vi "test-CoordinateSystem-checkTransform3dConvert.vi"(8 "COORDINATE_SYSTEM_TO":T1={"Rotation"={"Q_quaternion"={"R"=1.0, "V"=[0.0, 0.0, 0.0]}}}, 9 "COORDINATE_SYSTEM_FROM":T1={"Rotation"={"Q_quaternion"={"R"=1.0, "V"=[0.0, 0.0, 0.0]}}}, 10 "Transform3D_TO":T4={"TRANSLATION3D"={"X"=0.0, "Y"=0.0, "Z"=0.0}, "ROTATION3D"={"Q_quaternion"={"R"=1.0, "V"=[0.0, 0.0, 0.0]}}, "XF"=FALSE} {"TRANSLATION3D"."Z" format="%14.3f"; "TRANSLATION3D"."Y" format="%14.3f"; "TRANSLATION3D"."X" format="%14.3f"}, 11 "Transform3D_FROM":T4={"TRANSLATION3D"={"X"=0.0, "Y"=0.0, "Z"=0.0}, "ROTATION3D"={"Q_quaternion"={"R"=1.0, "V"=[0.0, 0.0, 0.0]}}, "XF"=FALSE} {"TRANSLATION3D"."Z" format="%14.3f"; "TRANSLATION3D"."Y" format="%14.3f"; "TRANSLATION3D"."X" format="%14.3f"}) -> (3 "All tests passed":bool)   [LabVIEW 2019]
uses:
  <vilib>/Rock Robotics/WPI/ThirdParty/JAS_Junk/TrajLib/TypeDef/TRANSFORM3D.ctl
  <vilib>/Rock Robotics/WPI/ThirdParty/JAS_Junk/TrajLib/TypeDef/TRANSLATION3D.ctl
  <vilib>/Rock Robotics/WPI/ThirdParty/JAS_Junk/TrajLib/TypeDef/ROTATION3D.ctl
  <vilib>/Rock Robotics/WPI/ThirdParty/JAS_Junk/TrajLib/TypeDef/QUATERNION.ctl
  <vilib>/Rock Robotics/WPI/ThirdParty/JAS_Junk/TrajLib/TypeDef/COORDINATE_SYSTEM.ctl
  <vilib>/Rock Robotics/WPI/ThirdParty/JAS_Junk/TrajLib/VI/Transform3d_Create_Trans3dRot3d.vi
  <vilib>/Rock Robotics/WPI/ThirdParty/JAS_Junk/TrajLib/VI/Rotation3d_Minus.vi
  <vilib>/Rock Robotics/WPI/ThirdParty/JAS_Junk/TrajLib/VI/Rotation3d_RotateBy.vi
  <vilib>/Rock Robotics/WPI/ThirdParty/JAS_Junk/TrajLib/VI/Translation3d_RotateBy.vi
  <vilib>/Rock Robotics/WPI/ThirdParty/JAS_Junk/TrajLib/VI/Rotation3d_GetQuaterion.vi
  <vilib>/Rock Robotics/WPI/ThirdParty/JAS_Junk/TrajLib/VI/Quaternion_Equals.vi
  <vilib>/Rock Robotics/WPI/ThirdParty/JAS_Junk/TrajLib/VI/Rotation3d_UnaryMinus.vi
  <vilib>/Rock Robotics/WPI/ThirdParty/JAS_Junk/TrajLib/VI/Rotation3d_Create_Quaternion.vi
  <vilib>/Rock Robotics/WPI/ThirdParty/JAS_Junk/TrajLib/VI/Quaternion_Times.vi
  <vilib>/Rock Robotics/WPI/ThirdParty/JAS_Junk/TrajLib/VI/Quaternion_New.vi
  <vilib>/Rock Robotics/WPI/ThirdParty/JAS_Junk/TrajLib/VI/Quaternion_Inverse.vi
  <vilib>/Rock Robotics/WPI/ThirdParty/JAS_Junk/TrajLib/VI/Quaternion_Get_All.vi
  <vilib>/Rock Robotics/WPI/ThirdParty/JAS_Junk/TrajLib/VI/Quaternion_Get_Vect.vi
  <vilib>/Rock Robotics/WPI/ThirdParty/JAS_Junk/TrajLib/VI/Quaternion_Get_W.vi
  <vilib>/Rock Robotics/WPI/ThirdParty/JAS_Junk/TrajLib/VI/Quaternion_Normalize.vi
  <vilib>/Rock Robotics/WPI/ThirdParty/JAS_Junk/TrajLib/VI/Quaternion_New_Default.vi
  <vilib>/Rock Robotics/WPI/ThirdParty/JAS_Junk/TrajLib/Trajectory_Library.lvlib
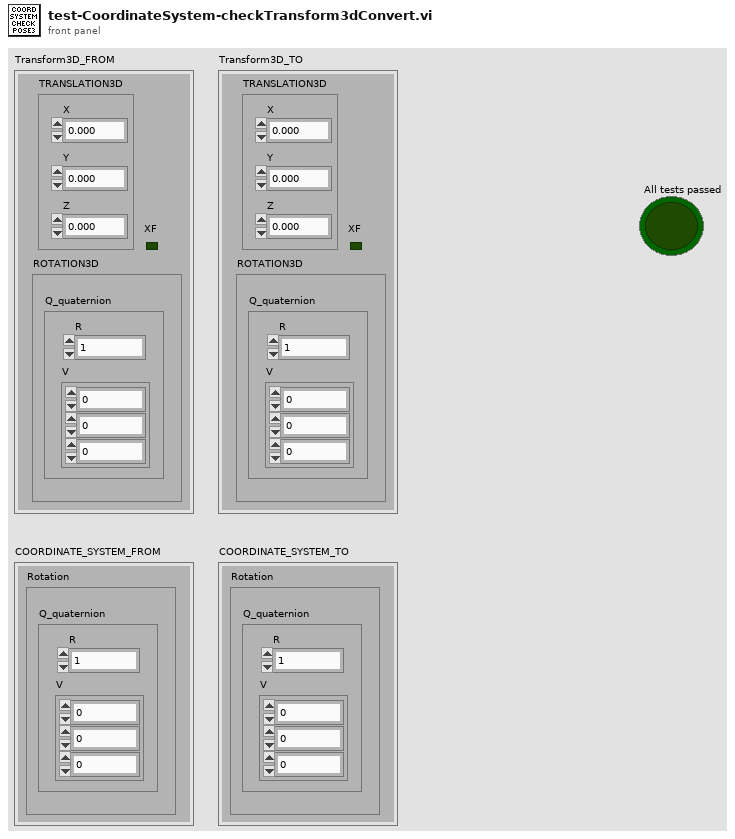
[diagram p1: front panel]
types:
  T1 = typedef "Trajectory_Library.lvlib/COORDINATE_SYSTEM.ctl" = cluster{"Rotation":T2}
  T2 = typedef "Trajectory_Library.lvlib/ROTATION3D.ctl" = cluster{"Q_quaternion":T3}
  T3 = typedef "Trajectory_Library.lvlib/QUATERNION.ctl" = cluster{"R":dbl, "V":dbl[]}
  T4 = typedef "Trajectory_Library.lvlib/TRANSFORM3D.ctl" = cluster{"TRANSLATION3D":T5, "ROTATION3D":T2, "XF":bool}
  T5 = typedef "Trajectory_Library.lvlib/TRANSLATION3D.ctl" = cluster{"X":dbl, "Y":dbl, "Z":dbl}
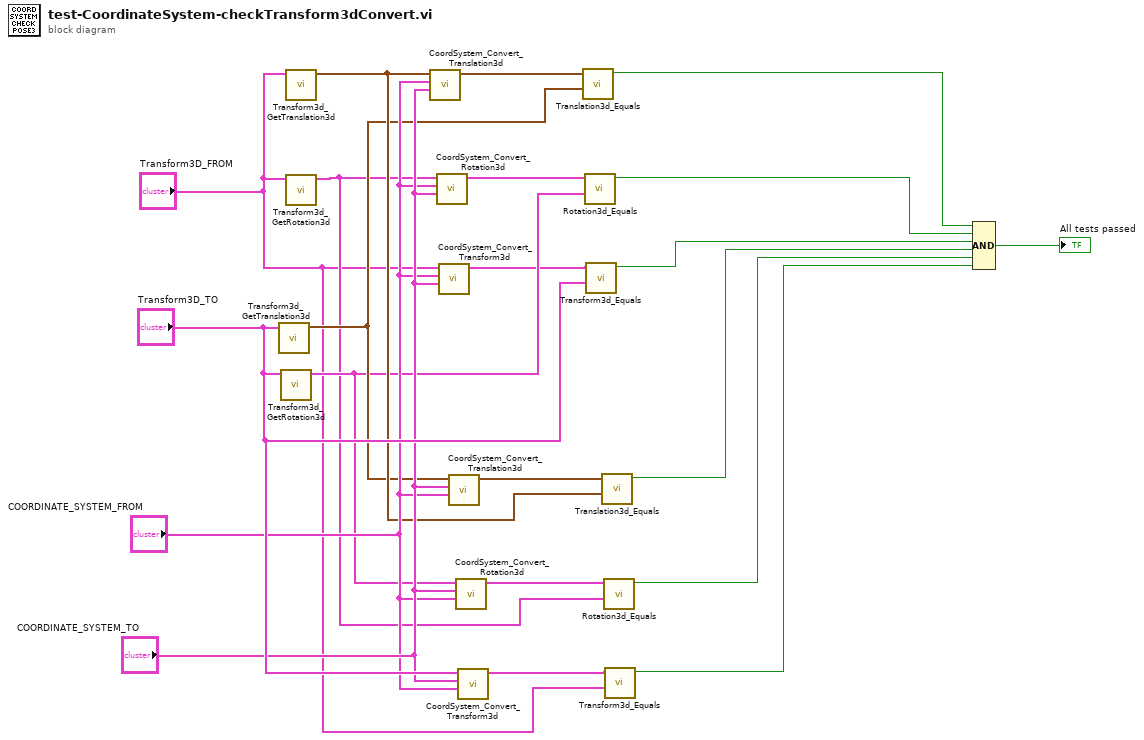
[diagram p0: block diagram]
diagram:
  n1 = call <vilib>:"Transform3d_GetTranslation3d.vi"("in Transform3d"="Transform3D_TO") -> ("Translation3d"=w11:T5)  [unwired: 10 in]
  n2 = call <vilib>:"Transform3d_GetRotation3d.vi"("in Transform3d"="Transform3D_TO") -> ("Rotation3d"=w10:T2)  [unwired: 10 in]
  n3 = call <vilib>:"Transform3d_GetTranslation3d.vi"("in Transform3d"="Transform3D_FROM") -> ("Translation3d"=w12:T5)  [unwired: 10 in]
  n4 = call <vilib>:"Transform3d_GetRotation3d.vi"("in Transform3d"="Transform3D_FROM") -> ("Rotation3d"=w9:T2)  [unwired: 10 in]
  n5 = call <vilib>:"CoordSystem_Convert_Translation3d.vi"("CoordSys To"="COORDINATE_SYSTEM_TO", "CoordSys From"="COORDINATE_SYSTEM_FROM", "in Translation3d"=w12) -> ("out Converted Translation3d"=w20:T5)  [unwired: 8 in]
  n6 = call <vilib>:"CoordSystem_Convert_Rotation3d.vi"("CoordSys To"="COORDINATE_SYSTEM_TO", "CoordSys From"="COORDINATE_SYSTEM_FROM", "in Rotation3d"=w9) -> ("out Converted Rotation3d"=w19:T2)  [unwired: 8 in]
  n7 = call <vilib>:"CoordSystem_Convert_Transform3d.vi"("CoordSys To"="COORDINATE_SYSTEM_TO", "CoordSys From"="COORDINATE_SYSTEM_FROM", "in Transform3d"="Transform3D_FROM") -> ("out Converted Transform3d"=w5:T4)  [unwired: 8 in]
  n8 = call <vilib>:"CoordSystem_Convert_Translation3d.vi"("CoordSys To"="COORDINATE_SYSTEM_FROM", "CoordSys From"="COORDINATE_SYSTEM_TO", "in Translation3d"=w11) -> ("out Converted Translation3d"=w18:T5)  [unwired: 8 in]
  n9 = call <vilib>:"CoordSystem_Convert_Rotation3d.vi"("CoordSys To"="COORDINATE_SYSTEM_FROM", "CoordSys From"="COORDINATE_SYSTEM_TO", "in Rotation3d"=w10) -> ("out Converted Rotation3d"=w17:T2)  [unwired: 8 in]
  n10 = call <vilib>:"CoordSystem_Convert_Transform3d.vi"("CoordSys To"="COORDINATE_SYSTEM_FROM", "CoordSys From"="COORDINATE_SYSTEM_TO", "in Transform3d"="Transform3D_TO") -> ("out Converted Transform3d"=w16:T4)  [unwired: 8 in]
  n11 = call <vilib>:"Translation3d_Equals.vi"("other Translation3d"=w11, "In Translation3d"=w20) -> ("Equals"=w7:bool)  [unwired: 9 in]
  n12 = call <vilib>:"Rotation3d_Equals.vi"("other Rotation3d"=w10, "in Rotation3d"=w19) -> ("Equals"=w6:bool)  [unwired: 9 in]
  n13 = call <vilib>:"Transform3d_Equals.vi"("otherTransform3d"="Transform3D_TO", "inTransform3d"=w5) -> ("Equals"=w4:bool)  [unwired: 9 in]
  n14 = call <vilib>:"Translation3d_Equals.vi"("other Translation3d"=w12, "In Translation3d"=w18) -> ("Equals"=w3:bool)  [unwired: 9 in]
  n15 = call <vilib>:"Rotation3d_Equals.vi"("other Rotation3d"=w9, "in Rotation3d"=w17) -> ("Equals"=w2:bool)  [unwired: 9 in]
  n16 = call <vilib>:"Transform3d_Equals.vi"("otherTransform3d"="Transform3D_FROM", "inTransform3d"=w16) -> ("Equals"=w1:bool)  [unwired: 9 in]
  n17 = Compound Arithmetic op=AND(w7, w6, w4, w3, w2, w1) -> (→"All tests passed":bool)
